vi "defPath.vi"(7 "Current VI path":path) -> (4 "settings path":path, 6 "database path":path)   [LabVIEW 2020, in "Sgraph_lib_V1.lvlib"]
doc: "Andre Koelewijn, 6 may 2017\n\nThis vi is used to set/get the default file path locations"
uses:
  Builds/Sgraph_lib_V1.lvlib
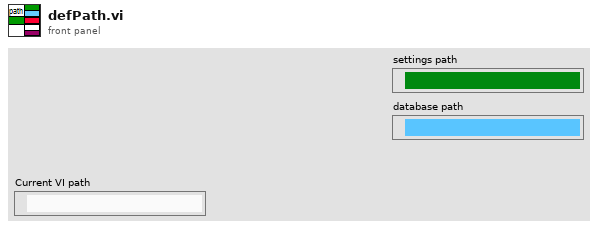
[diagram p1: front panel]
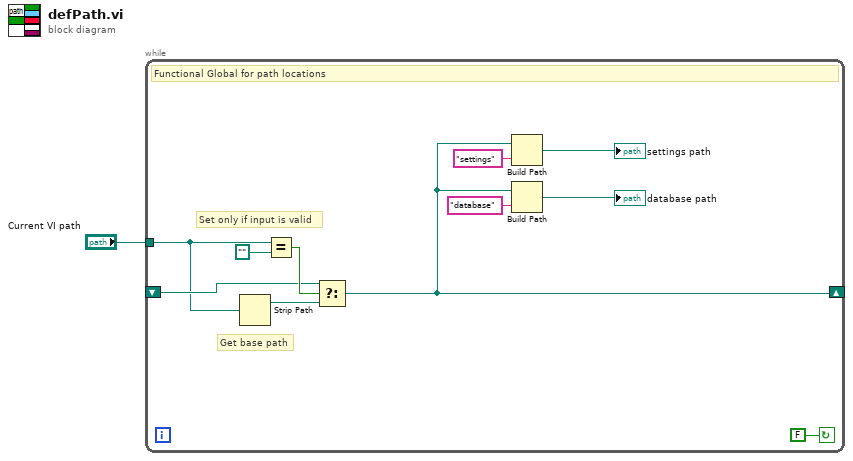
[diagram p0: block diagram]
diagram:
  n1 = while {
    shift-right: [w2] -> _
    shift-left: _ -> [w9]
    tunnel: "Current VI path" -> [w6]
    stop <- FALSE continue-if-true
    # "Get base path"
    # "Set only if input is valid"
    # "Functional Global for path locations"
    n2 = Strip Path(path=w6) -> (stripped path=w5:path)  [unwired: 1 out]
    n3 = Equal?(x=w6, y=path "") -> (x = y?=w10:bool)
    n4 = Select(t=w9, s=w10, f=w5) -> (s? t:f=w2:path)
    n5 = Build Path(base path=w2, name or relative path="settings") -> (appended path=→"settings path":path)
    n6 = Build Path(base path=w2, name or relative path="database") -> (appended path=→"database path":path)
  }
